vi "DataXML saveData.vi"(8 "error in (no error)":errorcluster, 11 "DataXML in":refnum<class "DataXML.lvclass">) -> (0 "error out":errorcluster, 3 "DataXML out":refnum<class "DataXML.lvclass">)   [LabVIEW 2018, in "DataXML.lvclass"]
uses:
  DataXML.lvclass
  DataXML.lvclass/DataXML.ctl
  <vilib>/xml/NI_XML.lvlib
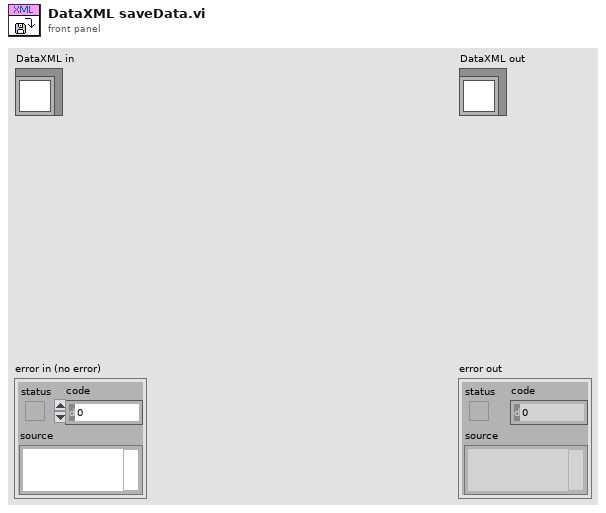
[diagram p1: front panel]
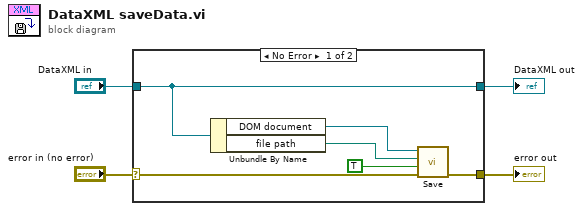
[diagram p0: block diagram]
diagram:
  n1 = case shown="No Error" "error in (no error)" {
    selector: "error in (no error)" -> [w6 w12]
    tunnel: [w5 w12] -> w3
    tunnel: [w10 w11] -> w1
    tunnel: "DataXML in" -> [w10 w11]
    frame No Error {
      n2 = Unbundle By Name(w10) -> ("DOM document"=w9:refnum<k20>, "file path"=w7:path)
      n3 = call <vilib>:"Save.vi"("error in (no error)"=w6, "overwrite file (True)"=TRUE, "XML file path"=w7, "DOM document in"=w9) -> ("error out"=w5:errorcluster)  [unwired: 5 in, 2 out]
    }
    frame Error {
    }
  }
  "error out" <- w3
  "DataXML out" <- w1
